vi "Data FIFO Probe (FXP).vi"(8 "Valid":bool=TRUE, 11 "Data":fxp<+/-,16,2>) -> (3 "Array":fxp<+/-,16,2>[](array[numeric]) format="%.14g")   [LabVIEW 2011]
doc: "This VI is used to probe Array of data on FPGA during simulation"
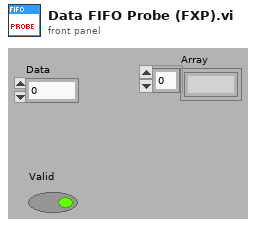
[diagram p1: front panel]
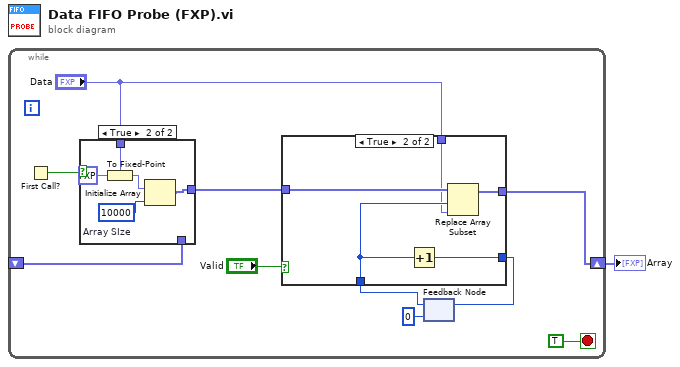
[diagram p0: block diagram]
diagram:
  n1 = while {
    shift-right: [w11] -> w1
    shift-left: _ -> [w9]
    stop <- TRUE stop-if-true
    n2 = First Call?() -> (First Call?: T/F=w7:bool)
    n3 = case shown="True" w7 {
      tunnel: [w19 w23] -> w10
      tunnel: w9 -> [w19 _]
      tunnel: "Data" -> [_ w20]
      frame False {
      }
      frame True {
        w24 = 10000  # Array SIze
        n4 = To Fixed-Point(fixed-point type=w20, number=fxp<+,1,1> 0.0) -> (fixed-point=w22:fxp<+/-,16,2>)
        n5 = Initialize Array(w22, w24) -> (w23:fxp<+/-,16,2>[])
      }
    }
    n6 = feedback #1(u32 0) -> (w4:u32)
    n7 = case shown="True" "Valid" {
      tunnel: [w13 w18] -> w11
      tunnel: w10 -> [w13 w17]
      tunnel: w4 -> [w12 w15]
      tunnel: [w12 w16] -> w3
      tunnel: "Data" -> [_ w14]
      frame False {
      }
      frame True {
        n8 = Increment(x=w15) -> (x+1=w16:u32)
        n9 = Replace Array Subset(array=w17, new element=w14, index=w15) -> (w18:fxp<+/-,16,2>[])
      }
    }
    n10 = feedback-in #1(w3) -> ()
  }
  "Array" <- w1
